vi "rad_Deploy Images with Progress.vi"(6 "Deployment Notifiers":T1[](array[typedef]), 7 "temp folder":path, 8 "error in (no error)":errorcluster, 9 "Target Config Options in":T4={"NumInBatch"=0, "Target Config Operation"=enum."No Config", "Target Name"="", "Increment Static IPs"=FALSE, "Change Target Name"=FALSE, "Primary NIC"={"MAC address"="", "IP Address Request Mode"=2, "IP address"="", "Subnet mask"="", "Gateway"="", "DNS server"=""}} {"Primary NIC"."IP Address Request Mode" items=["Static"=1, "DHCP/Link-Local"=2, "Link-Local Only"=4, "DHCP Only"=8]}, 10 "RT Deployment Targets in":T2[](array[typedef]) {"Primary NIC"."IP Address Request Mode" items=["Static"=1, "DHCP/Link-Local"=2, "Link-Local Only"=4, "DHCP Only"=8]}, 11 "image path":path) -> (0 "error out":errorcluster, 1 "Target Config Options out":T4={"NumInBatch"=0, "Target Config Operation"=enum."No Config", "Target Name"="", "Increment Static IPs"=FALSE, "Change Target Name"=FALSE, "Primary NIC"={"MAC address"="", "IP Address Request Mode"=2, "IP address"="", "Subnet mask"="", "Gateway"="", "DNS server"=""}} {"Primary NIC"."IP Address Request Mode" items=["Static"=1, "DHCP/Link-Local"=2, "Link-Local Only"=4, "DHCP Only"=8]}, 2 "Error Occurred":bool[](array[boolean]))   [LabVIEW 2021]
uses:
  TypeDefs/rad_Target Configuration Settings.ctl
  TypeDefs/rad_Target Configuration Operations.ctl
  Targets/TypeDefs/rad_Target Network Settings.ctl
  Targets/TypeDefs/rad_Target Information.ctl
  TypeDefs/rad_Application Image Properties.ctl
  TypeDefs/rad_FPGA Properties.ctl
  TypeDefs/rad_FPGA Flash Properties.ctl
  TypeDefs/rad_Deployment Notifiers.ctl
  TypeDefs/rad_Deployment Status Data Type.ctl
  TypeDefs/rad_Deployment Progress Data Type.ctl
  Targets/TypeDefs/rad_Initialize Access Types.ctl
  <vilib>/Utility/error.llb/Clear Errors.vi
  NI-Auth/rad_IPaddr and Password Global.vi
  rad_Globals.vi
  <vilib>/nisyscfg/Initialize Session.vi
  <vilib>/nisyscfg/Close (System).vi
  NI-Auth/rad_Open Session.vi
  <vilib>/nisyscfg/Set System Image (Folder).vi
  <vilib>/nisyscfg/nisyscfg.lvlib
panel:
  in  "State Variables":T10={"INI Modified"=FALSE, "Target Config. Options"={"NumInBatch"=0, "Target Config Operation"=enum."No Config", "Target Name"="", "Increment Static IPs"=FALSE, "Change Target Name"=FALSE, "Primary NIC"={"MAC address"="", "IP Address Request Mode"=2, "IP address"="", "Subnet mask"="", "Gateway"="", "DNS server"=""}}, "RT Deployment Targets"=[], "AppImage Properties"={"Name"="", "Version"="", "Time"=timestamp(0 s since 1904-01-01), "Description"="", "Key"="", "Chassis"="", "FPGA Properties"=[], "Model"="", "Retrieve"=[], "Deploy"=[], "Installed Software"=[]}, "Deployment Notifiers"=[], "Post-deployment access"=enum."Admin unless unlocked"} {"RT Deployment Targets"."Primary NIC"."IP Address Request Mode" items=["Static"=1, "DHCP/Link-Local"=2, "Link-Local Only"=4, "DHCP Only"=8]; "Target Config. Options"."Primary NIC"."IP Address Request Mode" items=["Static"=1, "DHCP/Link-Local"=2, "Link-Local Only"=4, "DHCP Only"=8]}
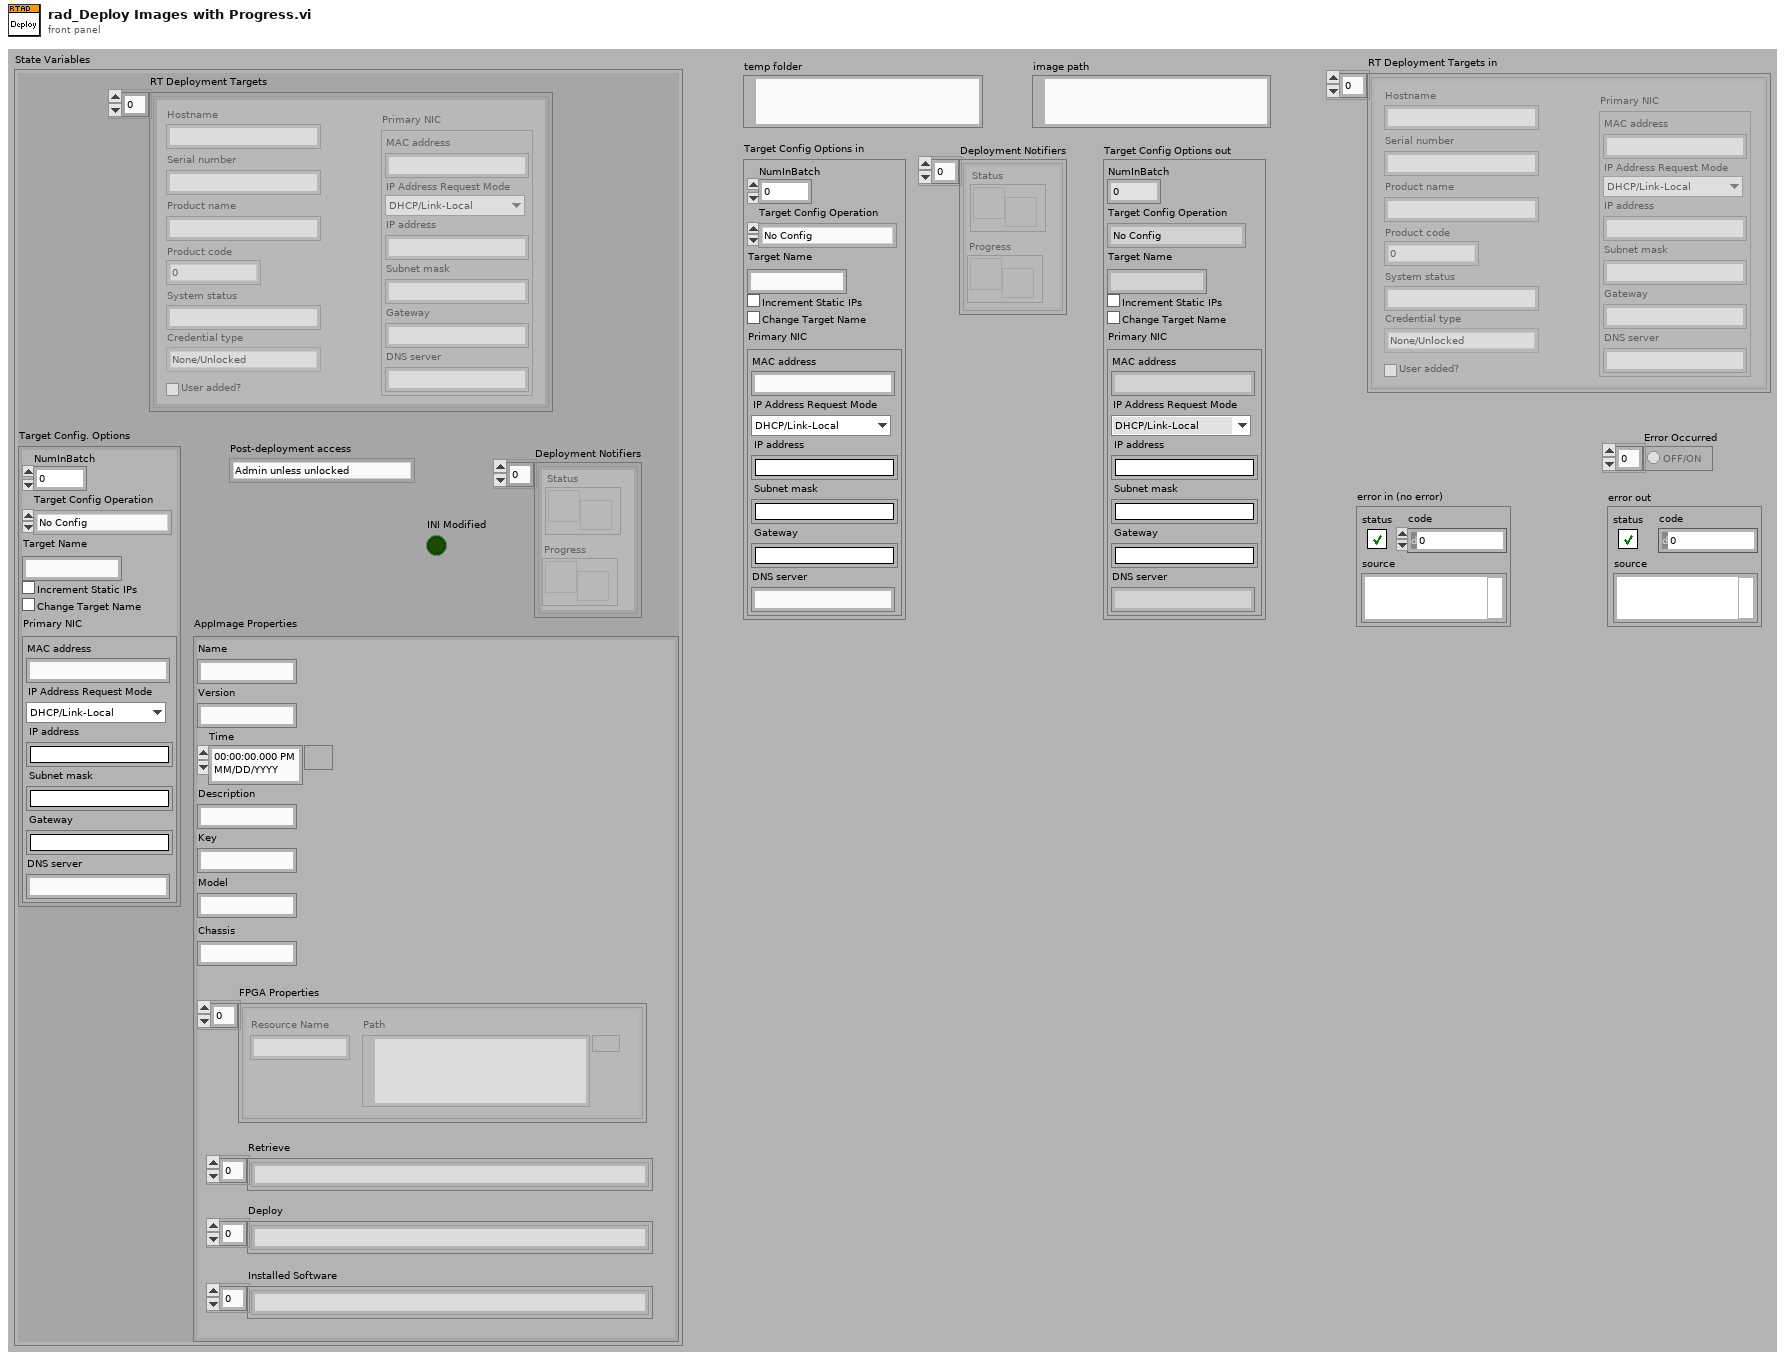
[diagram p1: front panel]
types:
  T1 = typedef "rad_Deployment Notifiers.ctl" = cluster{"Status":refnum<notifier>, "Progress":refnum<notifier>}
  T2 = typedef "rad_Target Information.ctl" = cluster{"Hostname":string, "Serial number":string, "Product name":string, "Product code":i32, "System status":string, "Credential type":enum16{"None/Unlocked", "FTP Password", "NIAuth Credentials"}, "User added?":bool, "Primary NIC":T3}
  T3 = typedef "rad_Target Network Settings.ctl" = cluster{"MAC address":string, "IP Address Request Mode":i32, "IP address":string, "Subnet mask":string, "Gateway":string, "DNS server":string}
  T4 = typedef "rad_Target Configuration Settings.ctl" = cluster{"NumInBatch":u32, "Target Config Operation":T5, "Target Name":string, "Increment Static IPs":bool, "Change Target Name":bool, "Primary NIC":T3}
  T5 = typedef "rad_Target Configuration Operations.ctl" = enum8{"No Config", "Image Config", "Static Config"}
  T6 = typedef "rad_Application Image Properties.ctl" = cluster{"Name":string, "Version":string, "Time":timestamp, "Description":string, "Key":string, "Chassis":string, "FPGA Properties":T7, "Model":string, "Retrieve":string[], "Deploy":string[], "Installed Software":string[]}
  T7 = typedef "rad_FPGA Properties.ctl" = T8[]
  T8 = typedef "rad_FPGA Flash Properties.ctl" = cluster{"Resource Name":string, "Path":path}
  T9 = typedef "rad_Initialize Access Types.ctl" = enum16{"Anonymous read-only", "Admin unless unlocked", "Admin always"}
  T10 = cluster{"INI Modified":bool, "Target Config. Options":T4, "RT Deployment Targets":T2[], "AppImage Properties":T6, "Deployment Notifiers":T1[], "Post-deployment access":T9}
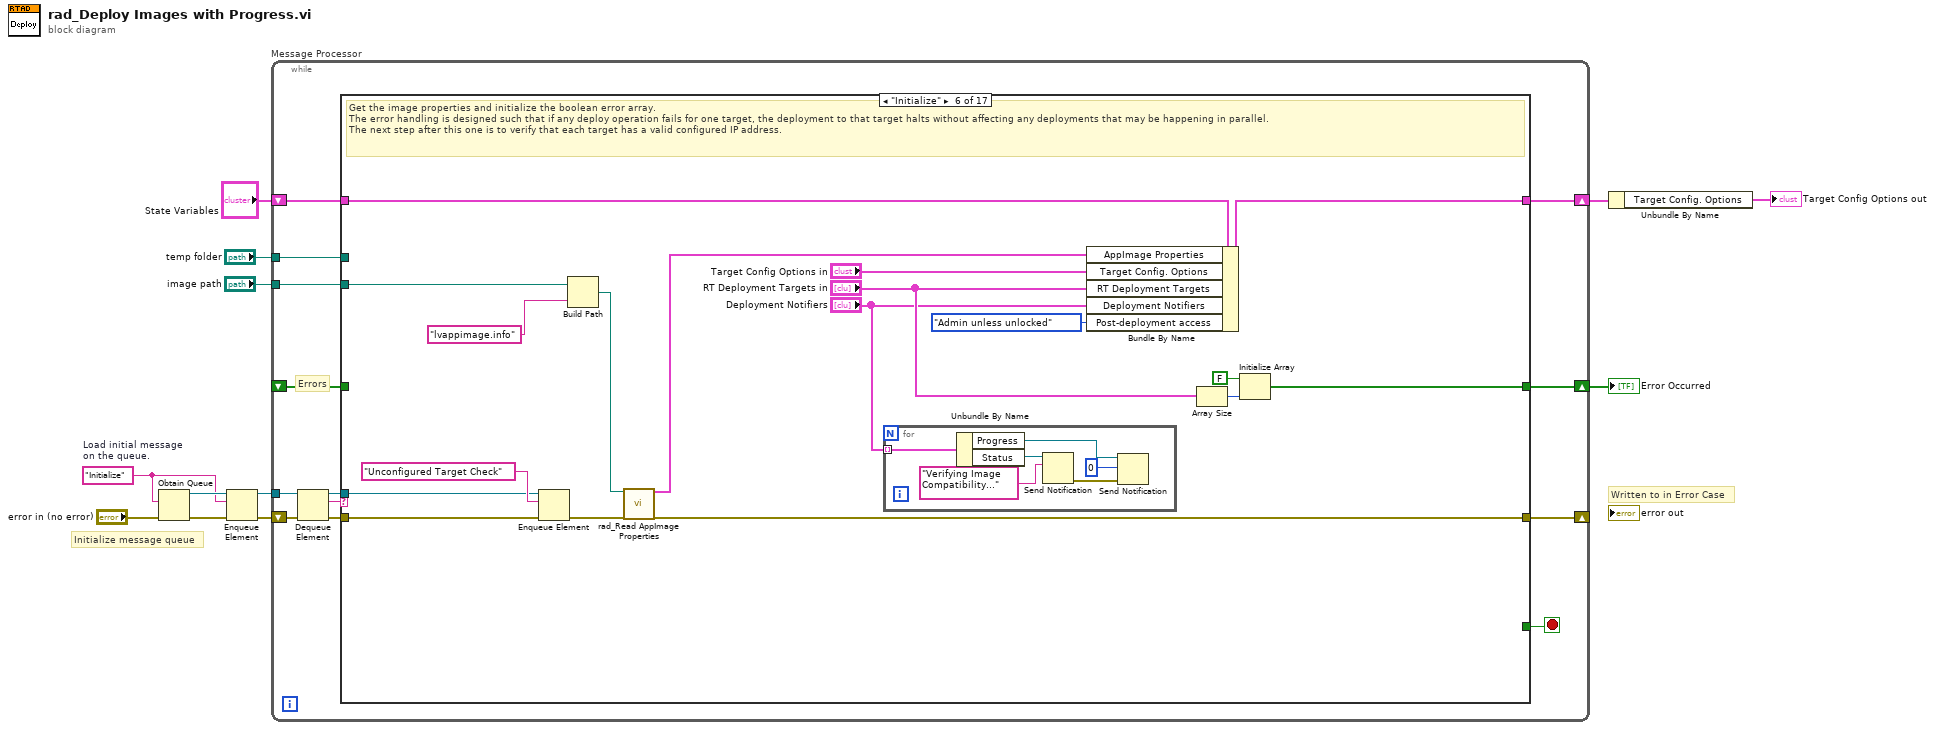
[diagram p0: block diagram]
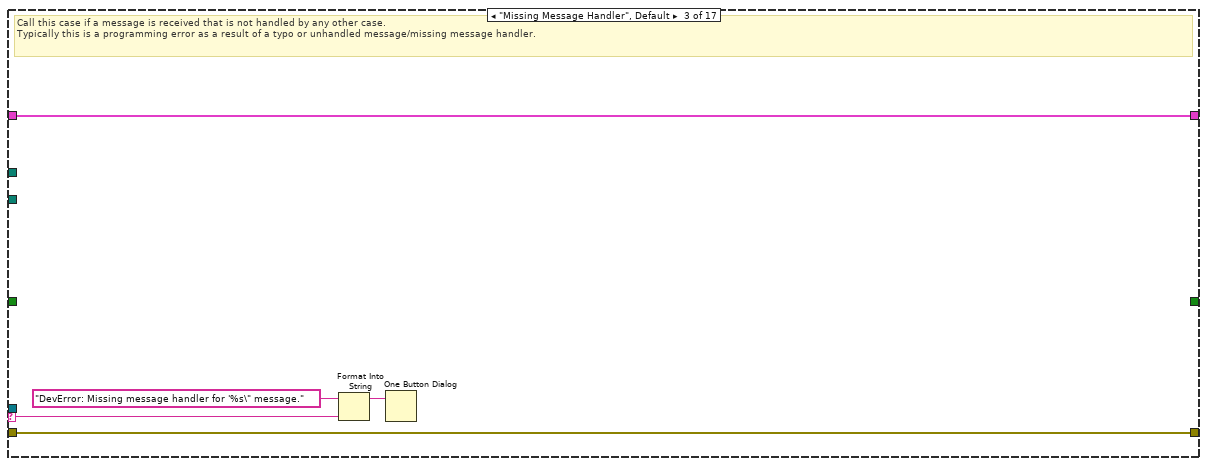
[diagram p4: hidden frame]
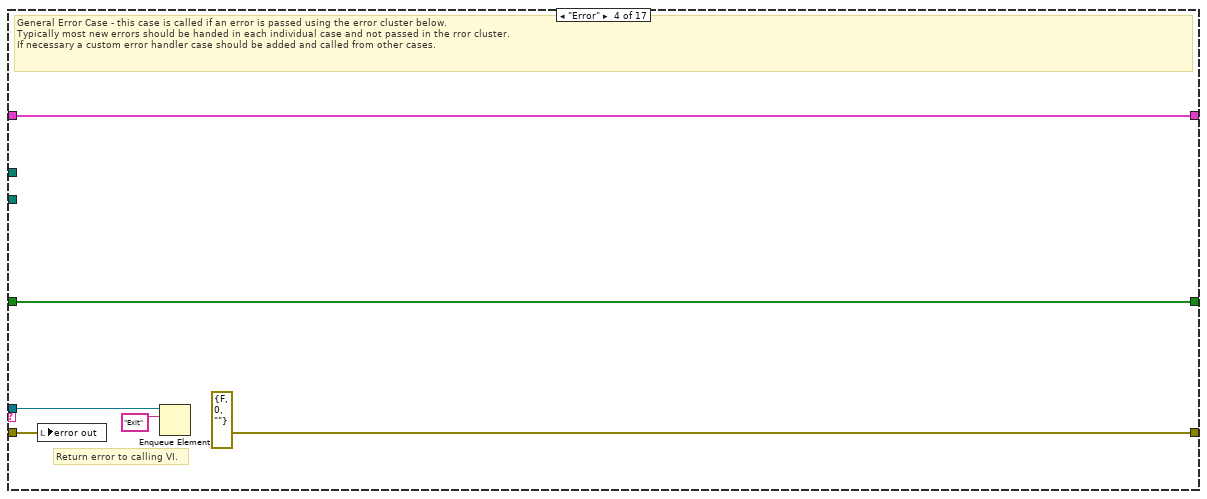
[diagram p5: hidden frame]
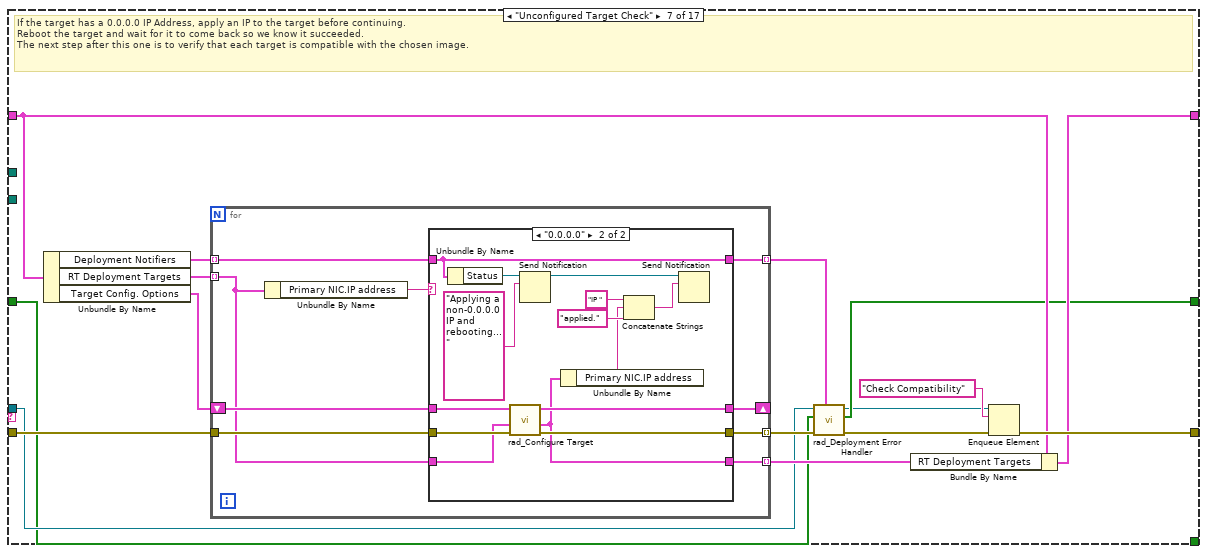
[diagram p7: hidden frame]
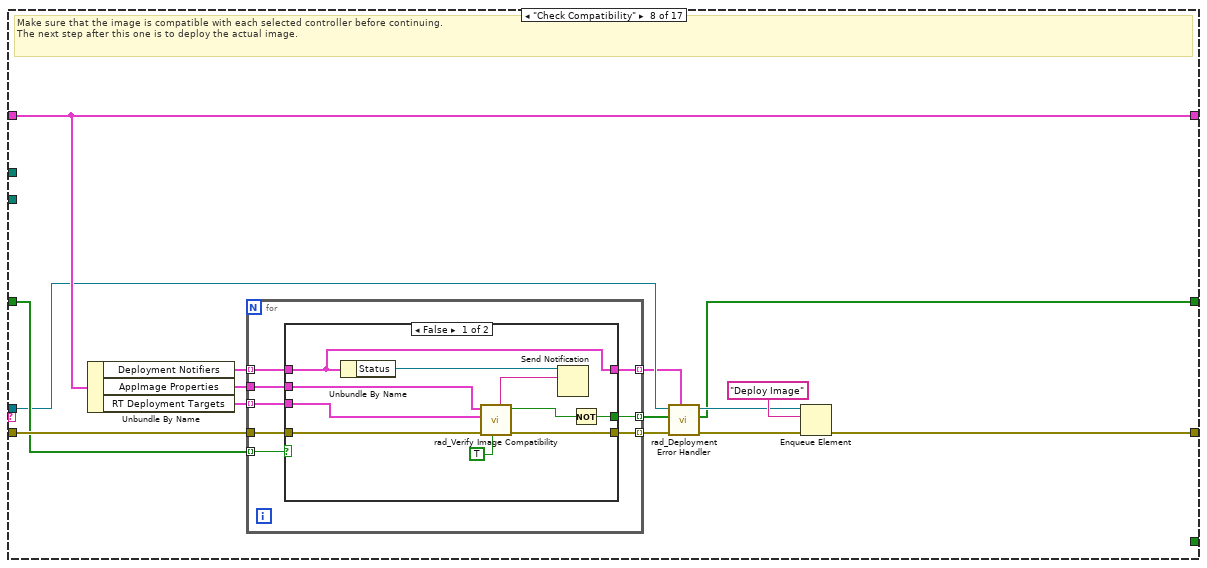
[diagram p9: hidden frame]
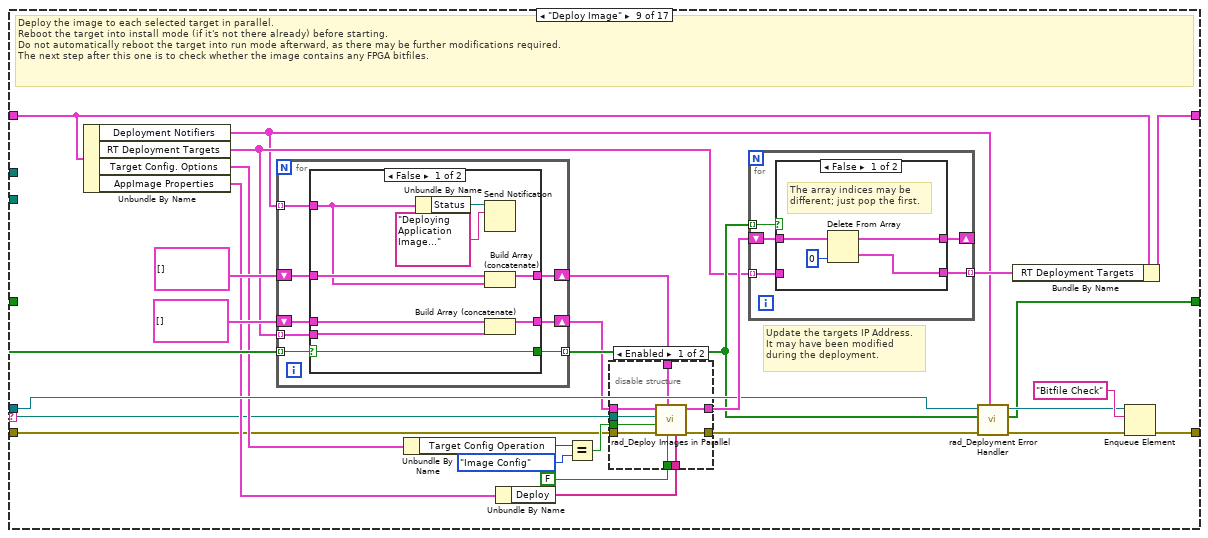
[diagram p11: hidden frame]
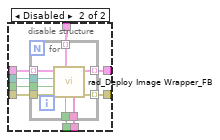
[diagram p12: hidden frame]
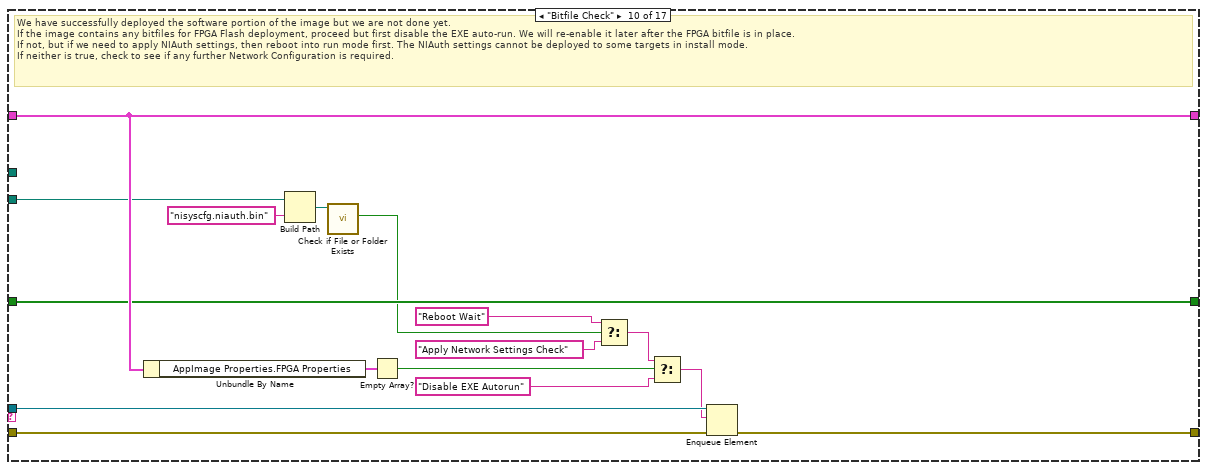
[diagram p15: hidden frame]
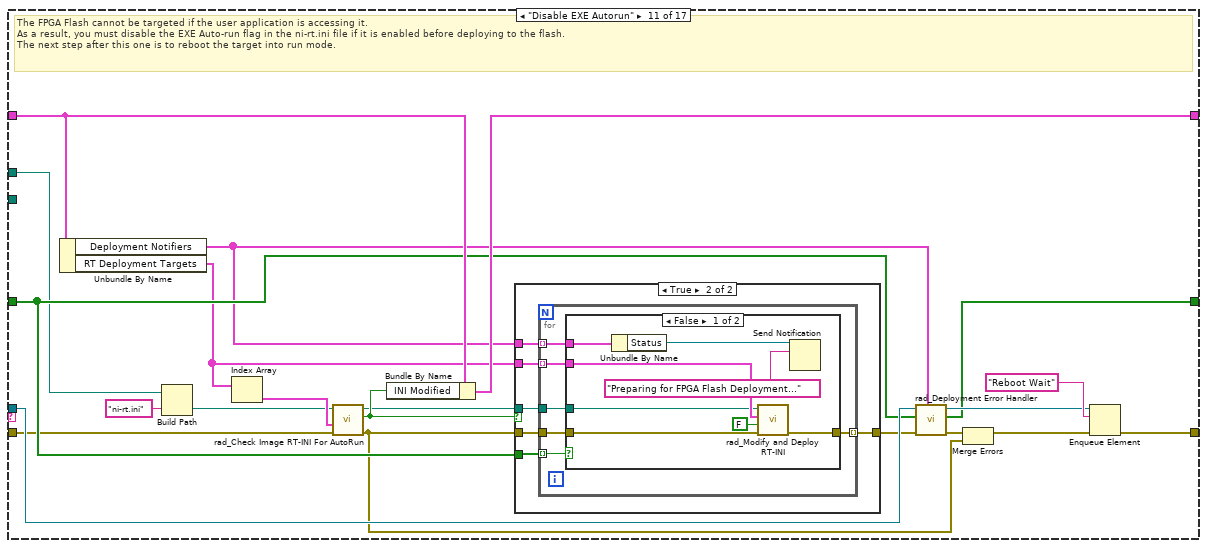
[diagram p16: hidden frame]
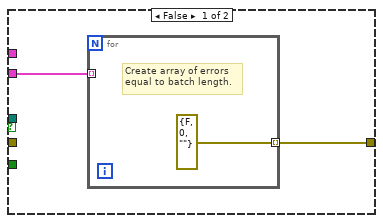
[diagram p17: hidden frame]
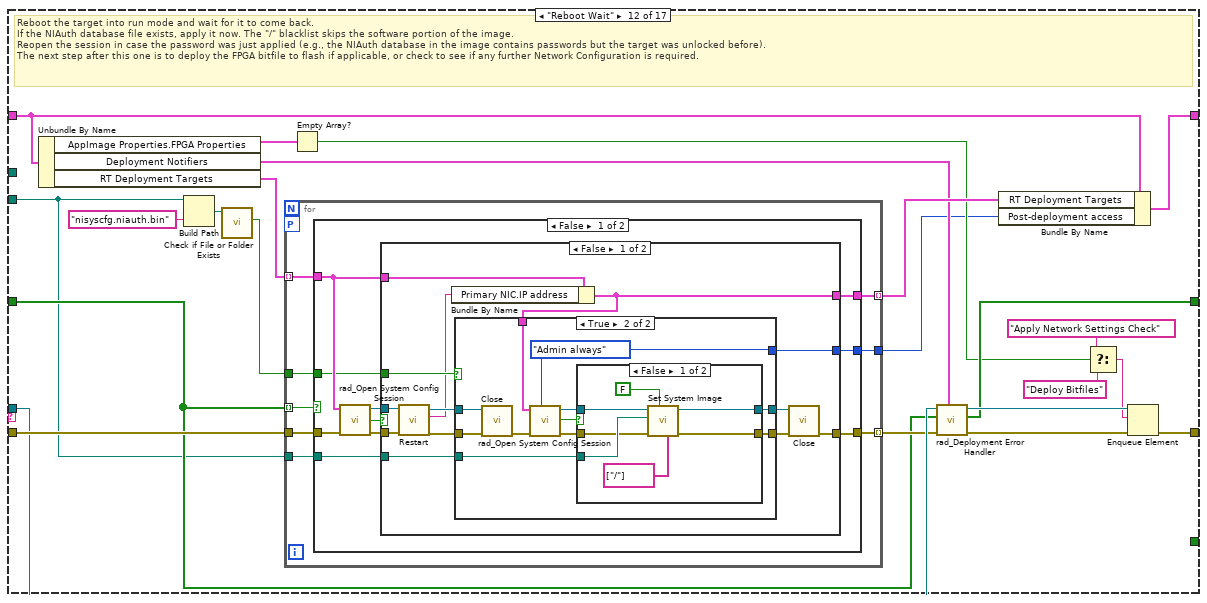
[diagram p19: hidden frame]
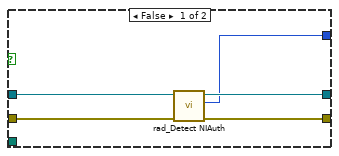
[diagram p20: hidden frame]
diagram:
  w1 = "Initialize"  # Load initial message on the queue.
  # "Written to in Error Case"
  # "Initialize message queue"
  n1 = Obtain Queue(element data type=w1, error in (no error)="error in (no error)") -> (queue out=w12:refnum<queue>, error out=w3:errorcluster)  [unwired: 3 in, 1 out]
  n2 = Enqueue Element(queue=w12, element=w1, error in (no error)=w3) -> (queue out=w4:refnum<queue>, error out=w2:errorcluster)  [unwired: 1 in, 1 out]
  n3 = while "Message Processor" {
    shift-left: w2 -> [w21]
    shift-right: [w14] -> _
    tunnel: w4 -> [w22]
    shift-left: "State Variables" -> [w25]
    shift-right: [w24] -> w9
    tunnel: "temp folder" -> [w18]
    tunnel: "image path" -> [w17]
    shift-right: [w15] -> w5
    shift-left: _ -> [w16]
    stop <- w13 stop-if-true
    # "Errors"
    n4 = Dequeue Element(queue=w22, error in (no error)=w21) -> (queue out=w23:refnum<queue>, element=w19:string, error out=w20:errorcluster)  [unwired: 1 in, 1 out]
    n5 = case shown="\"Initialize\"" w19 {
      selector: w19 -> [_ _ w33 _ _ _ _ _ _ _ _ _ _ _ _ _ _]
      tunnel: [w27 w30 w35 w41 w43 w60 w80 w124 w166 w246 w266 w311 w399 w439 w468 w515 w539] -> w24
      tunnel: w25 -> [w27 w30 w35 w41 w43 w61 w79 w124 w167 w246 w267 w313 w399 w439 w466 w515 w539]
      tunnel: w23 -> [_ _ _ w40 _ w45 w70 w117 w164 w247 w265 w309 w393 w436 w459 w522 w541]
      tunnel: w20 -> [w26 w29 w34 w37 w42 w50 w83 w119 w147 w245 w251 w314 w382 w427 w467 w524 w542]
      tunnel: [w26 w29 w34 errorcluster {"status"=FALSE, "code"=0, "source"=""} ("error out") w42 w51 w82 w125 w174 w248 w269 w316 w400 w438 w472 w526 w540] -> w14
      tunnel: w18 -> [_ _ _ _ _ _ _ _ _ _ w252 _ _ w428 _ _ _]
      tunnel: w17 -> [_ _ _ _ _ w49 _ _ w148 w240 _ w299 w381 _ _ _ _]
      tunnel: [_ w28 _ w36 _ w56 w74 w112 w159 w244 w262 w307 w392 w434 w457 w520 w537] -> w15
      tunnel: w16 -> [_ w28 _ w36 _ _ w68 w118 w172 w244 w259 w304 w388 w432 w452 w517 w537]
      tunnel: [_ _ _ _ _ _ _ _ _ _ _ _ _ _ _ _ TRUE] -> w13
      frame "---------- Framework Operations ----------" {
        # "Dummy case to add a seperator in the Case Structure menu."
      }
      frame "", "Idle" {
        # "Idle Case - this case is called after a Timeout on the Get Next Message from Queue VI, if no new messages are present on the queue.\nThis case can be used for housekeeping tasks such as updating the UI."
      }
      frame "Missing Message Handler", Default {
        # "Call this case if a message is received that is not handled by any other case.\nTypically this is a programming error as a result of a typo or unhandled message/missing message handler."
        n6 = Format Into String(format string="DevError: Missing message handler for '%s\" message." ("message"), w33) -> (resulting string=w31:string)  [unwired: 2 in, 1 out]
        n7 = One Button Dialog(message=w31) -> ()  [unwired: 2 out]
      }
      frame "Error" {
        # "Return error to calling VI."
        # "General Error Case - this case is called if an error is passed using the error cluster below.\nTypically most new errors should be handed in each individual case and not passed in the rror cluster.\nIf necessary a custom error handler case should be added and called from other cases."
        n8 = local write "error out"(w37) -> ()
        n9 = Enqueue Element(queue=w40, element="Exit") -> ()  [unwired: 2 in, 3 out]
      }
      frame "----------Application Operations ----------" {
        # "Dummy case to add a seperator in the Case Structure menu."
      }
      frame "Initialize" {
        # "Get the image properties and initialize the boolean error array. \nThe error handling is designed such that if any deploy operation fails for one target, the deployment to that target halts without affecting any deployments that may be happening in parallel. \nThe next step after this one is to verify that each target has a valid configured IP address."
        n10 = Enqueue Element(queue=w45, element="Unconfigured Target Check", error in (no error)=w50) -> (error out=w47:errorcluster)  [unwired: 1 in, 2 out]
        n11 = Build Path(base path=w49, name or relative path="lvappimage.info") -> (appended path=w52:path)
        n12 = call "rad_Read AppImage Properties.vi"("AppImage Properties Path"=w52, "error in (no error)"=w47) -> ("AppImage Properties"=w48:T6, "error out"=w51:errorcluster)  [unwired: 12 in, 4 out]
        n13 = for {
          tunnel: "Deployment Notifiers" -> [w66] mode=indexing
          n14 = Unbundle By Name(w66) -> ("Progress"=w64:refnum<notifier>, "Status"=w65:refnum<notifier>)
          n15 = Send Notification(notification="Verifying Image Compatibility...", notifier=w65) -> (error out=w63:errorcluster)  [unwired: 1 in, 1 out]
          n16 = Send Notification(notification=0, notifier=w64, error in (no error)=w63) -> ()  [unwired: 2 out]
        }
        n17 = Bundle By Name(cluster=w61, "AppImage Properties"=w48, "Target Config. Options"="Target Config Options in", "RT Deployment Targets"="RT Deployment Targets in", "Deployment Notifiers"="Deployment Notifiers", "Post-deployment access"=rad_Initialize_Access_Types."Admin unless unlocked") -> (w60:T10)
        n18 = Array Size(array="RT Deployment Targets in") -> (size(s)=w57:i32)
        n19 = Initialize Array(FALSE, w57) -> (w56:bool[])
      }
      frame "Unconfigured Target Check" {
        # "If the target has a 0.0.0.0 IP Address, apply an IP to the target before continuing. \nReboot the target and wait for it to come back so we know it succeeded. \nThe next step after this one is to verify that each target is compatible with the chosen image."
        n20 = Unbundle By Name(w79) -> ("Deployment Notifiers"=w78:T1[], "RT Deployment Targets"=w77:T2[], "Target Config. Options"=w76:T4)
        n21 = for {
          tunnel: w83 -> [w90]
          tunnel: [w92] -> w73 mode=indexing
          tunnel: w78 -> [w88] mode=indexing
          tunnel: w77 -> [w87] mode=indexing
          shift-right: [w89] -> _
          shift-left: w76 -> [w91]
          tunnel: [w86] -> w75 mode=indexing
          tunnel: [w85] -> w71 mode=indexing
          n22 = Unbundle By Name(w87) -> ("Primary NIC.IP address"=w84:string)
          n23 = case shown="\"0.0.0.0\"" w84 {
            tunnel: [w96 w102] -> w92
            tunnel: w91 -> [w94 w110]
            tunnel: w90 -> [w96 w103]
            tunnel: [w94 w109] -> w89
            tunnel: w88 -> [w93 w100]
            tunnel: w87 -> [w95 w99]
            tunnel: [w95 w98] -> w86
            tunnel: [w93 w100] -> w85
            frame Default {
            }
            frame "0.0.0.0" {
              n24 = Unbundle By Name(w100) -> ("Status"=w101:refnum<notifier>)
              n25 = call "rad_Configure Target.vi"("error in (no error)"=w103, "Target settings in"=w99, "Target Config Options in"=w110) -> ("error out"=w102:errorcluster, "Target settings out"=w98:T2, "Target Config Options out"=w109:T4)  [unwired: 6 in]
              n26 = Send Notification(notification="Applying a non-0.0.0.0 IP and rebooting...", notifier=w101) -> (notifier out=w107:refnum<notifier>)  [unwired: 1 in, 1 out]
              n27 = Unbundle By Name(w98) -> ("Primary NIC.IP address"=w97:string)
              n28 = Concatenate Strings("IP " ("notification"), w97, "applied." ("string")) -> (w104:string)
              n29 = Send Notification(notification=w104, notifier=w107) -> ()  [unwired: 1 in, 2 out]
            }
          }
        }
        n30 = call "rad_Deployment Error Handler.vi"("Deployment Notifiers"=w71, "error in (no error)"=w73, "Error Occurred"=w68, "Queue in"=w70) -> ("error out"=w72:errorcluster, "Error Occurred"=w74:bool[], "Queue out"=w69:refnum<queue>)  [unwired: 5 in]
        n31 = Bundle By Name(cluster=w79, "RT Deployment Targets"=w75) -> (w80:T10)
        n32 = Enqueue Element(queue=w69, element="Check Compatibility" ("Message Name"), error in (no error)=w72) -> (error out=w82:errorcluster)  [unwired: 1 in, 2 out]
      }
      frame "Check Compatibility" {
        # "Make sure that the image is compatible with each selected controller before continuing.\nThe next step after this one is to deploy the actual image."
        n33 = Unbundle By Name(w124) -> ("Deployment Notifiers"=w121:T1[], "AppImage Properties"=w120:T6, "RT Deployment Targets"=w122:T2[])
        n34 = for {
          tunnel: w122 -> [w131] mode=indexing
          tunnel: w121 -> [w129] mode=indexing
          tunnel: w120 -> [w133]
          tunnel: w119 -> [w132]
          tunnel: w118 -> [w130] mode=indexing
          tunnel: [w128] -> w115 mode=indexing
          tunnel: [w127] -> w116 mode=indexing
          tunnel: [w126] -> w114 mode=indexing
          n35 = case shown="False" w130 {
            selector: w130 -> [_ w146]
            tunnel: w133 -> [w143 _]
            tunnel: w132 -> [w142 w145]
            tunnel: w131 -> [w134 _]
            tunnel: w129 -> [w136 w144]
            tunnel: [w138 w146] -> w128
            tunnel: [w140 w145] -> w127
            tunnel: [w136 w144] -> w126
            frame False {
              n36 = Unbundle By Name(w136) -> ("Status"=w137:refnum<notifier>)
              n37 = call "rad_Verify Image Compatibility.vi"("Require Identical Chassis?"=TRUE, "error in (no error)"=w142, "Target address"=w134, "AppImage Properties"=w143) -> ("error out"=w140:errorcluster, "Compatible?"=w139:bool, "Status message"=w135:string)  [unwired: 5 in]
              n38 = Send Notification(notification=w135, notifier=w137) -> ()  [unwired: 1 in, 2 out]
              n39 = Not(x=w139) -> (.not. x?=w138:bool)
            }
            frame True {
            }
          }
        }
        n40 = call "rad_Deployment Error Handler.vi"("Deployment Notifiers"=w114, "error in (no error)"=w116, "Error Occurred"=w115, "Queue in"=w117) -> ("error out"=w111:errorcluster, "Error Occurred"=w112:bool[], "Queue out"=w113:refnum<queue>)  [unwired: 5 in]
        n41 = Enqueue Element(queue=w113, element="Deploy Image" ("t"), error in (no error)=w111) -> (error out=w125:errorcluster)  [unwired: 1 in, 2 out]
      }
      frame "Deploy Image" {
        # "Update the targets IP Address.\nIt may have been modified\nduring the deployment."
        # "Deploy the image to each selected target in parallel. \nReboot the target into install mode (if it's not there already) before starting.\nDo not automatically reboot the target into run mode afterward, as there may be further modifications required. \nThe next step after this one is to check whether the image contains any FPGA bitfiles."
        n42 = Unbundle By Name(w167) -> ("Deployment Notifiers"=w156:T1[], "RT Deployment Targets"=w157:T2[], "Target Config. Options"=w152:T4, "AppImage Properties"=w151:T6)
        n43 = for {
          tunnel: w156 -> [w219] mode=indexing
          tunnel: w172 -> [w220] mode=indexing
          tunnel: [w218] -> w162 mode=indexing
          tunnel: w157 -> [w217] mode=indexing
          shift-right: [w216] -> w169
          shift-left: T1[] [] ("Deployment Notifiers") -> [w215]
          shift-right: [w214] -> w149
          shift-left: T2[] [] -> [w213]
          n44 = case shown="False" w220 {
            selector: w220 -> [w228 w232]
            tunnel: w219 -> [w223 _]
            tunnel: [w228 w232] -> w218
            tunnel: w217 -> [w221 _]
            tunnel: [w227 w230] -> w216
            tunnel: w215 -> [w226 w230]
            tunnel: [w225 w231] -> w214
            tunnel: w213 -> [w224 w231]
            frame False {
              n45 = Unbundle By Name(w223) -> ("Status"=w222:refnum<notifier>)
              n46 = Send Notification(notification="Deploying Application Image...", notifier=w222) -> ()  [unwired: 1 in, 2 out]
              n47 = Build Array (concatenate)(w226, w223) -> (w227:T1[])
              n48 = Build Array (concatenate)(w224, w221) -> (w225:T2[])
            }
            frame True {
            }
          }
        }
        n49 = Unbundle By Name(w152) -> ("Target Config Operation"=w155:T5)
        n50 = Unbundle By Name(w151) -> ("Deploy"=w150:string[])
        n51 = Equal?(x=w155, y=rad_Target_Configuration_Operations."Image Config" ("x")) -> (x = y?=w153:bool)
        n52 = disable-structure shown="Enabled" {
          disable-tunnel: FALSE ("restart after imaging? (T)") -> [w183 w185]
          disable-tunnel: w169 -> [w182 w188]
          disable-tunnel: [w181 w187] -> w168
          disable-tunnel: [w180 w186] -> w163
          disable-tunnel: w153 -> [w179 w189]
          disable-tunnel: w150 -> [w178 w184]
          disable-tunnel: w149 -> [w177 w191]
          disable-tunnel: w148 -> [w176 w190]
          disable-tunnel: w147 -> [w175 w192]
          frame Enabled {
            n53 = call "rad_Deploy Images in Parallel.vi"("Deploy"=w178, "restart after imaging (T)"=w183, "Deployment Notifiers"=w182, "error in (no error)"=w175, "apply primary NIC from image (F)"=w179, "image file path in"=w176, "Target addresses in"=w177) -> ("Errors Out"=w180:errorcluster[], "Target addresses out"=w181:T2[])  [unwired: 2 in, 1 out]
          }
          frame Disabled {
            n54 = for {
              tunnel: w192 -> [w201]
              tunnel: w191 -> [w200] mode=indexing
              tunnel: w190 -> [w199]
              tunnel: w189 -> [w198]
              tunnel: w188 -> [w197] mode=indexing
              tunnel: [w196] -> w187 mode=indexing
              tunnel: [w195] -> w186 mode=indexing
              tunnel: w185 -> [w194]
              tunnel: w184 -> [w193]
              n55 = call "rad_Deploy Image Wrapper_FB.vi"("Deploy"=w193, "restart after imaging (T)"=w194, "Deployment Notifiers"=w197, "error in (no error)"=w201, "apply primary NIC from image (F)"=w198, "image file path"=w199, "Target settings in"=w200) -> ("error out"=w195:errorcluster, "Target settings out"=w196:T2)  [unwired: 2 in, 1 out]
            }
          }
        }
        n56 = for {
          tunnel: w162 -> [w206] mode=indexing
          tunnel: w157 -> [w204] mode=indexing
          shift-right: [w202] -> _
          shift-left: w168 -> [w205]
          tunnel: [w203] -> w165 mode=indexing
          n57 = case shown="False" w206 {
            tunnel: w205 -> [w210 w212]
            tunnel: w204 -> [_ w211]
            tunnel: [w208 w211] -> w203
            tunnel: [w209 w212] -> w202
            frame False {
              # "The array indices may be\ndifferent; just pop the first."
              n58 = Delete From Array(array=w210, index=0) -> (deleted portion=w208:T2, array with subset deleted=w209:T2[])  [unwired: 1 in]
            }
            frame True {
              # "An error happened earlier,\nso keep the existing address."
            }
          }
        }
        n59 = call "rad_Deployment Error Handler.vi"("Deployment Notifiers"=w156, "error in (no error)"=w163, "Error Occurred"=w162, "Queue in"=w164) -> ("error out"=w160:errorcluster, "Error Occurred"=w159:bool[], "Queue out"=w161:refnum<queue>)  [unwired: 5 in]
        n60 = Bundle By Name(cluster=w167, "RT Deployment Targets"=w165) -> (w166:T10)
        n61 = Enqueue Element(queue=w161, element="Bitfile Check" ("Message Name"), error in (no error)=w160) -> (error out=w174:errorcluster)  [unwired: 1 in, 2 out]
      }
      frame "Bitfile Check" {
        # "We have successfully deployed the software portion of the image but we are not done yet.\nIf the image contains any bitfiles for FPGA Flash deployment, proceed but first disable the EXE auto-run. We will re-enable it later after the FPGA bitfile is in place.\nIf not, but if we need to apply NIAuth settings, then reboot into run mode first. The NIAuth settings cannot be deployed to some targets in install mode.\nIf neither is true, check to see if any further Network Configuration is required."
        n62 = Unbundle By Name(w246) -> ("AppImage Properties.FPGA Properties"=w243:T7)
        n63 = Build Path(base path=w240, name or relative path="nisyscfg.niauth.bin") -> (appended path=w238:path)
        n64 = call <vilib>:"Check if File or Folder Exists.vi"("path"=w238) -> ("file or folder exists?"=w235:bool)  [unwired: 8 in, 2 out]
        n65 = Empty Array?(array=w243) -> (empty?=w241:bool)
        n66 = Select(t="Reboot Wait" ("Title"), s=w235, f="Apply Network Settings Check" ("Title")) -> (s? t:f=w236:string)
        n67 = Select(t=w236, s=w241, f="Disable EXE Autorun" ("Title")) -> (s? t:f=w237:string)
        n68 = Enqueue Element(queue=w247, element=w237, error in (no error)=w245) -> (error out=w248:errorcluster)  [unwired: 1 in, 2 out]
      }
      frame "Disable EXE Autorun" {
        # "The FPGA Flash cannot be targeted if the user application is accessing it.\nAs a result, you must disable the EXE Auto-run flag in the ni-rt.ini file if it is enabled before deploying to the flash.\nThe next step after this one is to reboot the target into run mode."
        n69 = Unbundle By Name(w267) -> ("Deployment Notifiers"=w258:T1[], "RT Deployment Targets"=w257:T2[])
        n70 = Build Path(base path=w252, name or relative path="ni-rt.ini") -> (appended path=w250:path)
        n71 = Index Array(array=w257) -> (element=w253:T2)  [unwired: 1 in]
        n72 = call "rad_Check Image RT-INI For AutoRun.vi"("error in (no error)"=w251, "target settings"=w253, "temp folder"=w250) -> ("error out"=w256:errorcluster, "Run at Startup?"=w255:bool, "temp folder out"=w254:path)  [unwired: 6 in]
        n73 = Bundle By Name(cluster=w267, "INI Modified"=w255) -> (w266:T10)
        n74 = case shown="True" w255 {
          tunnel: [w270 w277] -> w263
          tunnel: w256 -> [_ w278]
          tunnel: w257 -> [w271 w276]
          tunnel: w259 -> [_ w275]
          tunnel: w258 -> [_ w274]
          tunnel: w254 -> [_ w273]
          frame False {
            n75 = for {
              tunnel: w271 -> [_] mode=indexing
              tunnel: [errorcluster {"status"=FALSE, "code"=0, "source"=""} ("error out")] -> w270 mode=indexing
              # "Create array of errors\nequal to batch length."
            }
          }
          frame True {
            n76 = for {
              tunnel: w278 -> [w284]
              tunnel: [w283] -> w277 mode=indexing
              tunnel: w276 -> [w282] mode=indexing
              tunnel: w275 -> [w281] mode=indexing
              tunnel: w274 -> [w280] mode=indexing
              tunnel: w273 -> [w279]
              n77 = case shown="False" w281 {
                tunnel: w284 -> [w286 w293]
                tunnel: [w291 w293] -> w283
                tunnel: w282 -> [w287 _]
                tunnel: w280 -> [w289 _]
                tunnel: w279 -> [w285 _]
                frame False {
                  n78 = Unbundle By Name(w289) -> ("Status"=w288:refnum<notifier>)
                  n79 = call "rad_Modify and Deploy RT-INI.vi"("error in (no error)"=w286, "Run at Startup?"=FALSE, "Target settings"=w287, "temp folder"=w285) -> ("error out"=w291:errorcluster)  [unwired: 7 in]
                  n80 = Send Notification(notification="Preparing for FPGA Flash Deployment...", notifier=w288) -> ()  [unwired: 1 in, 2 out]
                }
                frame True {
                }
              }
            }
          }
        }
        n81 = call "rad_Deployment Error Handler.vi"("Deployment Notifiers"=w258, "error in (no error)"=w263, "Error Occurred"=w259, "Queue in"=w265) -> ("error out"=w261:errorcluster, "Error Occurred"=w262:bool[], "Queue out"=w264:refnum<queue>)  [unwired: 5 in]
        n82 = Merge Errors(w261, w256) -> (w260:errorcluster)
        n83 = Enqueue Element(queue=w264, element="Reboot Wait" ("Message Name"), error in (no error)=w260) -> (error out=w269:errorcluster)  [unwired: 1 in, 2 out]
      }
      frame "Reboot Wait" {
        # "Reboot the target into run mode and wait for it to come back.\nIf the NIAuth database file exists, apply it now. The \"/\" blacklist skips the software portion of the image.\nReopen the session in case the password was just applied (e.g., the NIAuth database in the image contains passwords but the target was unlocked before).\nThe next step after this one is to deploy the FPGA bitfile to flash if applicable, or check to see if any further Network Configuration is required."
        n84 = Unbundle By Name(w313) -> ("AppImage Properties.FPGA Properties"=w303:T7, "Deployment Notifiers"=w310:T1[], "RT Deployment Targets"=w315:T2[])
        n85 = Build Path(base path=w299, name or relative path="nisyscfg.niauth.bin") -> (appended path=w301:path)
        n86 = call <vilib>:"Check if File or Folder Exists.vi"("path"=w301) -> ("file or folder exists?"=w300:bool)  [unwired: 8 in, 2 out]
        n87 = for {
          tunnel: w315 -> [w322] mode=indexing
          tunnel: w314 -> [w324]
          tunnel: [w323] -> w305 mode=indexing
          tunnel: [w321] -> w312 mode=indexing
          tunnel: w304 -> [w320] mode=indexing
          workers-P: _ -> [_]
          tunnel: w300 -> [w319]
          tunnel: w299 -> [w318]
          tunnel: [w317] -> w294
          n88 = case shown="False" w320 {
            tunnel: w324 -> [w334 w377]
            tunnel: [w327 w377] -> w323
            tunnel: w322 -> [w330 w378]
            tunnel: [w329 w378] -> w321
            tunnel: w319 -> [w328 _]
            tunnel: w318 -> [w326 _]
            tunnel: [w325 rad_Initialize_Access_Types."Admin unless unlocked" ("Access requirement (admin unless unlocked)")] -> w317
            frame False {
              n89 = call "rad_Open System Config Session.vi"("error in (no error)"=w334, "Target settings"=w330) -> ("error out"=w331:errorcluster, "Cancelled"=w333:bool, "Session out"=w332:refnum<k21>)  [unwired: 6 in, 1 out]
              n90 = case shown="False" w333 {
                tunnel: w332 -> [w346 _]
                tunnel: w331 -> [w347 w374]
                tunnel: w330 -> [w338 w375]
                tunnel: [w336 w375] -> w329
                tunnel: w328 -> [w345 _]
                tunnel: [w340 w374] -> w327
                tunnel: w326 -> [w339 _]
                tunnel: [w335 rad_Initialize_Access_Types."Admin unless unlocked" ("Access requirement (admin unless unlocked)")] -> w325
                frame False {
                  n91 = call <vilib>:"Restart.vi"("error in (no error)"=w347, "Session in"=w346) -> ("error out"=w343:errorcluster, "New IP Address"=w337:string, "Session out"=w344:refnum<k21>)  [unwired: 7 in]
                  n92 = Bundle By Name(cluster=w338, "Primary NIC.IP address"=w337) -> (w336:T2)
                  n93 = case shown="True" w345 {
                    tunnel: w344 -> [w352 w359]
                    tunnel: w343 -> [w351 w360]
                    tunnel: [w349 w362] -> w342
                    tunnel: [w350 w363] -> w341
                    tunnel: w339 -> [_ w361]
                    tunnel: [w348 w354] -> w335
                    tunnel: w336 -> [_ w353]
                    frame False {
                      n94 = call "rad_Detect NIAuth.vi"("error in (no error)"=w351, "Session in"=w352) -> ("error out"=w350:errorcluster, "Post-deployment access"=w348:T9, "Session out"=w349:refnum<k21>)  [unwired: 7 in]
                    }
                    frame True {
                      w354 = rad_Initialize_Access_Types."Admin always" ("Access requirement (admin unless unlocked)")
                      n95 = call-poly <vilib>:"Close.vi"("error in (no error)"=w360, "Session in"=w359) -> ("error out"=w358:errorcluster)  [unwired: 9 in]
                      n96 = call "rad_Open System Config Session.vi"("Access requirement (admin unless unlocked)"=w354, "error in (no error)"=w358, "Target settings"=w353) -> ("error out"=w355:errorcluster, "Cancelled"=w357:bool, "Session out"=w356:refnum<k21>)  [unwired: 5 in, 1 out]
                      n97 = case shown="False" w357 {
                        tunnel: [w370 w371] -> w363
                        tunnel: [w369 w372] -> w362
                        tunnel: w361 -> [w366 _]
                        tunnel: w356 -> [w365 w372]
                        tunnel: w355 -> [w364 w371]
                        frame False {
                          n98 = call-poly <vilib>:"Set System Image.vi"("File and Directory Blacklist"=string[] ["/"], "Restart Automatically (T)"=FALSE ("restart automatically (T)"), "error in (no error)"=w364, "Source Folder"=w366, "Session in"=w365) -> ("error out"=w370:errorcluster, "Session out"=w369:refnum<k21>)  [unwired: 5 in]
                        }
                        frame True {
                        }
                      }
                    }
                  }
                  n99 = call-poly <vilib>:"Close.vi"("error in (no error)"=w341, "Session in"=w342) -> ("error out"=w340:errorcluster)  [unwired: 9 in]
                }
                frame True {
                }
              }
            }
            frame True {
            }
          }
        }
        n100 = Empty Array?(array=w303) -> (empty?=w295:bool)
        n101 = call "rad_Deployment Error Handler.vi"("Deployment Notifiers"=w310, "error in (no error)"=w305, "Error Occurred"=w304, "Queue in"=w309) -> ("error out"=w306:errorcluster, "Error Occurred"=w307:bool[], "Queue out"=w308:refnum<queue>)  [unwired: 5 in]
        n102 = Bundle By Name(cluster=w313, "RT Deployment Targets"=w312, "Post-deployment access"=w294) -> (w311:T10)
        n103 = Select(t="Apply Network Settings Check" ("Message Name"), s=w295, f="Deploy Bitfiles" ("Message Name")) -> (s? t:f=w296:string)
        n104 = Enqueue Element(queue=w308, element=w296, error in (no error)=w306) -> (error out=w316:errorcluster)  [unwired: 1 in, 2 out]
      }
      frame "Deploy Bitfiles" {
        # "We have at least one FPGA bitfile and the EXE is not running, so deploy the bitfile to flash now.\nThe next step after this one is to re-enable the EXE Autorun flag in the ni-rt.ini file if it was modified, or check to see if any further Network Configuration is required."
        n105 = Unbundle By Name(w399) -> ("Deployment Notifiers"=w380:T1[], "Post-deployment access"=w379:T9, "RT Deployment Targets"=w394:T2[], "AppImage Properties.FPGA Properties"=w386:T7, "INI Modified"=w395:bool)
        n106 = List Folder(path=w381, pattern="*.lvbitx", error in=w382) -> (filenames=w384:string[])  [unwired: 1 in, 3 out]
        n107 = for {
          tunnel: w381 -> [w403]
          tunnel: w384 -> [w402] mode=indexing
          tunnel: [w401] -> w383 mode=indexing
          n108 = Build Path(base path=w403, name or relative path=w402) -> (appended path=w401:path)
        }
        n109 = for {
          tunnel: w386 -> [w411]
          tunnel: w383 -> [w410]
          tunnel: [w409] -> w391 mode=indexing
          tunnel: w394 -> [w408] mode=indexing
          tunnel: w382 -> [w407]
          tunnel: w380 -> [w406] mode=indexing
          tunnel: w388 -> [w405] mode=indexing
          tunnel: w379 -> [w404]
          n110 = case shown="False" w405 {
            tunnel: w411 -> [w422 _]
            tunnel: w410 -> [w421 _]
            tunnel: [w417 errorcluster {"status"=FALSE, "code"=0, "source"=""} ("error out")] -> w409
            tunnel: w408 -> [w413 _]
            tunnel: w407 -> [w420 _]
            tunnel: w406 -> [w415 _]
            tunnel: w404 -> [w412 _]
            frame False {
              n111 = Unbundle By Name(w415) -> ("Status"=w414:refnum<notifier>)
              n112 = Send Notification(notification="Deploying to FPGA Flash...", notifier=w414) -> (notifier out=w418:refnum<notifier>)  [unwired: 1 in, 1 out]
              n113 = call "rad_Deploy All Bitfiles.vi"("Access requirement"=w412, "error in (no error)"=w420, "FPGA Properties"=w422, "Unzipped files"=w421, "Target settings in"=w413) -> ("error out"=w417:errorcluster)  [unwired: 6 in]
              n114 = Send Notification(notification="FPGA Flash Deployed.", notifier=w418, error in (no error)=w417) -> ()  [unwired: 2 out]
            }
            frame True {
            }
          }
        }
        n115 = call "rad_Deployment Error Handler.vi"("Deployment Notifiers"=w380, "error in (no error)"=w391, "Error Occurred"=w388, "Queue in"=w393) -> ("error out"=w390:errorcluster, "Error Occurred"=w392:bool[], "Queue out"=w387:refnum<queue>)  [unwired: 5 in]
        n116 = Select(t="Enable EXE Autorun" ("Title"), s=w395, f="Apply Network Settings Check") -> (s? t:f=w397:string)
        n117 = Merge Errors(w390, w382) -> (w389:errorcluster)
        n118 = Enqueue Element(queue=w387, element=w397, error in (no error)=w389) -> (error out=w400:errorcluster)  [unwired: 1 in, 2 out]
      }
      frame "Enable EXE Autorun" {
        # "Re-enable the startup EXE in the ni-rt.ini file if it was disabled previously.\nThe next step after this one is to check to see if any further Network Configuration is required."
        n119 = Build Path(base path=w428, name or relative path="ni-rt.ini") -> (appended path=w425:path)
        n120 = Unbundle By Name(w439) -> ("Deployment Notifiers"=w426:T1[], "RT Deployment Targets"=w429:T2[])
        n121 = for {
          tunnel: w425 -> [w444]
          tunnel: w427 -> [w443]
          tunnel: w429 -> [w441] mode=indexing
          tunnel: [w442] -> w435 mode=indexing
          tunnel: w432 -> [w440] mode=indexing
          n122 = case shown="False" w440 {
            tunnel: w444 -> [w445 _]
            tunnel: w443 -> [w446 _]
            tunnel: [w448 errorcluster {"status"=FALSE, "code"=0, "source"=""} ("error out")] -> w442
            tunnel: w441 -> [w447 _]
            frame False {
              n123 = call "rad_Modify and Deploy RT-INI.vi"("error in (no error)"=w446, "Run at Startup?"=TRUE, "Target settings"=w447, "temp folder"=w445) -> ("error out"=w448:errorcluster)  [unwired: 7 in]
            }
            frame True {
            }
          }
        }
        n124 = call "rad_Deployment Error Handler.vi"("Deployment Notifiers"=w426, "error in (no error)"=w435, "Error Occurred"=w432, "Queue in"=w436) -> ("error out"=w431:errorcluster, "Error Occurred"=w434:bool[], "Queue out"=w433:refnum<queue>)  [unwired: 5 in]
        n125 = Merge Errors(w431, w427) -> (w430:errorcluster)
        n126 = Enqueue Element(queue=w433, element="Apply Network Settings Check" ("Message Name"), error in (no error)=w430) -> (error out=w438:errorcluster)  [unwired: 1 in, 2 out]
      }
      frame "Apply Network Settings Check" {
        # "If we need to apply static network settings to each target, do so now.\nReboot each target into run mode and wait for it to come back so we know it succeeded.\nOtherwise, reboot each target into run mode but do not bother waiting for it to come back."
        n127 = Unbundle By Name(w466) -> ("Deployment Notifiers"=w454:T1[], "RT Deployment Targets"=w463:T2[], "Target Config. Options"=w464:T4)
        n128 = Unbundle By Name(w464) -> ("Target Config Operation"=w465:T5)
        n129 = Or Array Elements(Boolean array=w452) -> (logical OR=w453:bool)
        n130 = Equal?(x=w465, y=rad_Target_Configuration_Operations."Static Config") -> (x = y?=w469:bool)
        n131 = case shown="True" w469 {
          tunnel: w467 -> [_ w488]
          tunnel: [w475 w487] -> w458
          tunnel: [w479 w486] -> w462
          tunnel: w464 -> [w479 w485]
          tunnel: w463 -> [w478 w484]
          tunnel: [w478 w483] -> w461
          tunnel: w454 -> [w474 w482]
          tunnel: w453 -> [_ w481]
          tunnel: [w474 w480] -> w451
          frame False {
            n132 = Array Size(array=w478) -> (size(s)=w477:i32)
            n133 = Initialize Array(errorcluster {"status"=FALSE, "code"=0, "source"=""} ("error out"), w477) -> (w475:errorcluster[])
          }
          frame True {
            n134 = for {
              tunnel: w488 -> [w497]
              tunnel: [w496] -> w487 mode=indexing
              tunnel: w484 -> [w493] mode=indexing
              shift-right: [w495] -> w486
              shift-left: w485 -> [w494]
              tunnel: [w492] -> w483 mode=indexing
              tunnel: w482 -> [w491] mode=indexing
              tunnel: w481 -> [w490]
              tunnel: [w489] -> w480 mode=indexing
              n135 = case shown="False" w490 {
                tunnel: w497 -> [w506 w514]
                tunnel: [w501 w514] -> w496
                tunnel: [w510 w513] -> w495
                tunnel: w494 -> [w509 w513]
                tunnel: w493 -> [w499 w512]
                tunnel: [w498 w512] -> w492
                tunnel: w491 -> [w500 w511]
                tunnel: [w500 w511] -> w489
                frame False {
                  n136 = Unbundle By Name(w500) -> ("Status"=w507:refnum<notifier>)
                  n137 = Send Notification(notification="Applying deployment network settings...", notifier=w507, error in (no error)=w506) -> (error out=w505:errorcluster)  [unwired: 1 out]
                  n138 = call "rad_Configure Target.vi"("error in (no error)"=w505, "Target settings in"=w499, "Target Config Options in"=w509) -> ("error out"=w502:errorcluster, "Target settings out"=w498:T2, "Target Config Options out"=w510:T4)  [unwired: 6 in]
                  n139 = Unbundle By Name(w500) -> ("Status"=w504:refnum<notifier>)
                  n140 = Send Notification(notification="Network settings applied.", notifier=w504, error in (no error)=w502) -> (error out=w501:errorcluster)  [unwired: 1 out]
                }
                frame True {
                }
              }
            }
          }
        }
        n141 = Bundle By Name(cluster=w466, "RT Deployment Targets"=w461, "Target Config. Options"=w462) -> (w468:T10)
        n142 = call "rad_Deployment Error Handler.vi"("Deployment Notifiers"=w451, "error in (no error)"=w458, "Error Occurred"=w452, "Queue in"=w459) -> ("error out"=w456:errorcluster, "Error Occurred"=w457:bool[], "Queue out"=w455:refnum<queue>)  [unwired: 5 in]
        n143 = Select(t="Exit", s=w469, f="Reboot No Wait") -> (s? t:f=w460:string)
        n144 = Enqueue Element(queue=w455, element=w460, error in (no error)=w456) -> (error out=w472:errorcluster)  [unwired: 1 in, 2 out]
      }
      frame "Reboot No Wait" {
        # "We're done imaging the target, put it back into run mode."
        n145 = Unbundle By Name(w515) -> ("Deployment Notifiers"=w516:T1[], "RT Deployment Targets"=w525:T2[])
        n146 = for {
          tunnel: w525 -> [w528] mode=indexing
          tunnel: w524 -> [w530]
          tunnel: [w529] -> w519 mode=indexing
          tunnel: w517 -> [w527] mode=indexing
          workers-P: _ -> [_]
          n147 = case shown="False" w527 {
            tunnel: w530 -> [w533 w535]
            tunnel: [w532 w535] -> w529
            tunnel: w528 -> [w531 _]
            frame False {
              n148 = call "rad_Reboot (IP) Wrapper.vi"("error in (no error)"=w533, "wait for restart? (F)"=FALSE, "Target settings in"=w531) -> ("error out"=w532:errorcluster)  [unwired: 7 in, 1 out]
            }
            frame True {
            }
          }
        }
        n149 = call "rad_Deployment Error Handler.vi"("Deployment Notifiers"=w516, "error in (no error)"=w519, "Error Occurred"=w517, "Queue in"=w522) -> ("error out"=w518:errorcluster, "Error Occurred"=w520:bool[], "Queue out"=w521:refnum<queue>)  [unwired: 5 in]
        n150 = Enqueue Element(queue=w521, element="Exit" ("Message Name"), error in (no error)=w518) -> (error out=w526:errorcluster)  [unwired: 1 in, 2 out]
      }
      frame "Exit" {
        # "Nothing left to do!"
        n151 = Release Queue(queue=w541, error in (no error)=w542) -> (error out=w540:errorcluster)  [unwired: 1 in, 2 out]
        n152 = Unbundle By Name(w539) -> ("Deployment Notifiers"=w538:T1[])
        n153 = for {
          tunnel: w538 -> [w544] mode=indexing
          tunnel: w537 -> [w543] mode=indexing
          n154 = case shown="False" w543 {
            tunnel: w544 -> [w545 _]
            frame False {
              n155 = Unbundle By Name(w545) -> ("Status"=w546:refnum<notifier>)
              n156 = Send Notification(notification="Deployment Complete!", notifier=w546) -> ()  [unwired: 1 in, 2 out]
            }
            frame True {
            }
          }
        }
      }
    }
  }
  "Error Occurred" <- w5
  n157 = Unbundle By Name(w9) -> ("Target Config. Options"=→"Target Config Options out":T4)
